vi "Configure Rx.vi"(0 "niUsrpRio Session":T3={"FPGA Interface"=refnum, "RIO Interface Number"=0, "Data Clock Rate"=0, "FPGA Data Clock Rate"=0, "Global Settings Register Bus"=refnum, "Radio 0 Settings Register Bus"=refnum, "Radio 1 Settings Register Bus"=refnum, "Radio Settings Bus Semaphore"=refnum, "DB Queues"=[], "Characterization Data Valid?"=FALSE, "EEPROM Header"={"Checksum"=0, "Product Code"=0, "Hardware Current Version"=0, "Hardware Oldest Compatible Version"=0, "EEPROM Map Current Version"=0, "EEPROM Map Oldest Compatible Version"=0, "User Password"="", "Pointer to Factory Header"=0, "Pointer to User Header"=0, "Recommended Interval"=0, "Number of Reserved Bytes"=9, "Number of Daughterboards"=0, "Daughterboard IDs"=[], "Daughterboard Serial Numbers"=[]}, "Device Data Header"={"Checksum"=0, "Number of Channels"=0, "Number of Gain Settings"=[], "Pointer to Characterization Data"=[], "Number of Reserved Bytes"=27, "Number of Frequencies"=[]}, "EEPROM Characterization Header"={"Checksum"=0, "Date"=timestamp(0 s since 1904-01-01), "Temperature"=0.0, "Misc. Info"="", "Pointer to Device Data Header"=0, "Number of Reserved Bytes"=28}, "Characterization Data"=[], "FPGA Current Version"=0, "FPGA Oldest Compatible Version"=0, "Fixed Logic Current Version"=0, "Fixed Logic Oldest Compatible Version"=0, "FPGA Radio Settings Bus Current Version"=0, "FPGA Radio Settings Bus Oldest Compatible Version"=0, "FPGA Board Config Current Version"=0, "FPGA Board Config Oldest Compatible Version"=0, "Daughterboard Clock Rate"=0, "daughterboard configuration session handles"=[]} {"Daughterboard Clock Rate" format="%#.3pHz"; "FPGA Data Clock Rate" format="%#.3pHz"; "Data Clock Rate" format="%#.3pHz"; "Characterization Data"."Frequencies [Hz]" format="%#_6p"; "EEPROM Characterization Header"."Pointer to Device Data Header" format="%x"; "EEPROM Characterization Header"."Checksum" format="%x"; "Device Data Header"."Pointer to Characterization Data" format="%x"; "Device Data Header"."Checksum" format="%x"; "EEPROM Header"."Pointer to User Header" format="%x"; "EEPROM Header"."Pointer to Factory Header" format="%x"; "EEPROM Header"."Product Code" format="%x"; "EEPROM Header"."Checksum" format="%x"}, 5 "rx config":T2={"channel configuration"=[], "transfer mode"=enum."Finite", "sample rate"=10000000.0, "number of samples"=8192, "start trigger"=enum."Immediate"} {"channel configuration"."channel configuration"."frequency" format="%#.3pHz"; "channel configuration"."channel configuration"."lo frequency" format="%#.3pHz"; "channel configuration"."channel configuration"."level" format="%#_gdBm"; "sample rate" format="%#.3pS/s"}, 7 "rx.data sink":enum16{"SFP Port 0", "SFP Port 1", "Host"}(ring)=enum."Host", 11 "error in":errorcluster) -> (4 "niUsrpRio Session (out)":T3 {"Daughterboard Clock Rate" format="%#.3pHz"; "FPGA Data Clock Rate" format="%#.3pHz"; "Data Clock Rate" format="%#.3pHz"; "Characterization Data"."Frequencies [Hz]" format="%#_6p"; "EEPROM Characterization Header"."Pointer to Device Data Header" format="%x"; "EEPROM Characterization Header"."Checksum" format="%x"; "Device Data Header"."Pointer to Characterization Data" format="%x"; "Device Data Header"."Checksum" format="%x"; "EEPROM Header"."Pointer to User Header" format="%x"; "EEPROM Header"."Pointer to Factory Header" format="%x"; "EEPROM Header"."Product Code" format="%x"; "EEPROM Header"."Checksum" format="%x"}, 6 "rx.enabled channels":string[](array[string]), 8 "vertical range":dbl[](array[numeric]) format="%#.3pVpp", 14 "rx.coerced configurations":T12 {"coerced sample rates" format="%#.3pS/s"; "coerced levels" format="%#.3gdBm"; "coerced lo frequencies" format="%#.3pHz"; "coerced frequencies" format="%#.3pHz"}, 15 "error out":errorcluster)   [LabVIEW 2018]
uses:
  <instrlib>/niUsrpRio/Config/v1/Host/Public/niUsrpRio Session.ctl
  <instrlib>/_niInstr/Register Bus/v0/Host/Public/Register Bus Session.ctl
  <instrlib>/_niInstr/Register Bus/v0/Host/Private/Session Data.ctl
  <instrlib>/niUsrpRio/Config/v1/Host/Private/DB Queue Reference.ctl
  <instrlib>/niUsrpRio/Config/v1/Host/Private/Daughterboard Data.ctl
  <instrlib>/niUsrpRio/Config/v1/Host/Private/ATR state data.ctl
  <instrlib>/niUsrpRio/Config/v1/Host/Private/Antenna Configuration.ctl
  <instrlib>/niUsrpRio/Config/v1/Host/Private/CPLD Power Mode.ctl
  <instrlib>/niUsrpRio/Config/v1/Host/Public/EEPROM Header.ctl
  <instrlib>/niUsrpRio/Config/v1/Host/Public/EEPROM Device Data Header.ctl
  <instrlib>/niUsrpRio/Config/v1/Host/Public/EEPROM Characterization Header.ctl
  <instrlib>/niUsrpRio/Config/v1/Host/Public/Characterization Data.ctl
  <instrlib>/niUsrpRio/Config/v1/Host/Public/IQ Imbalance.ctl
  Start Trigger.ctl
  Configure Signal (Level).vi
  <instrlib>/niUsrpRio/Config/v1/Host/niUsrpRio Config v1 Host.lvlib
  <instrlib>/_niInstr/Register Bus/v0/Host/niInstr Register Bus v0 Host.lvlib
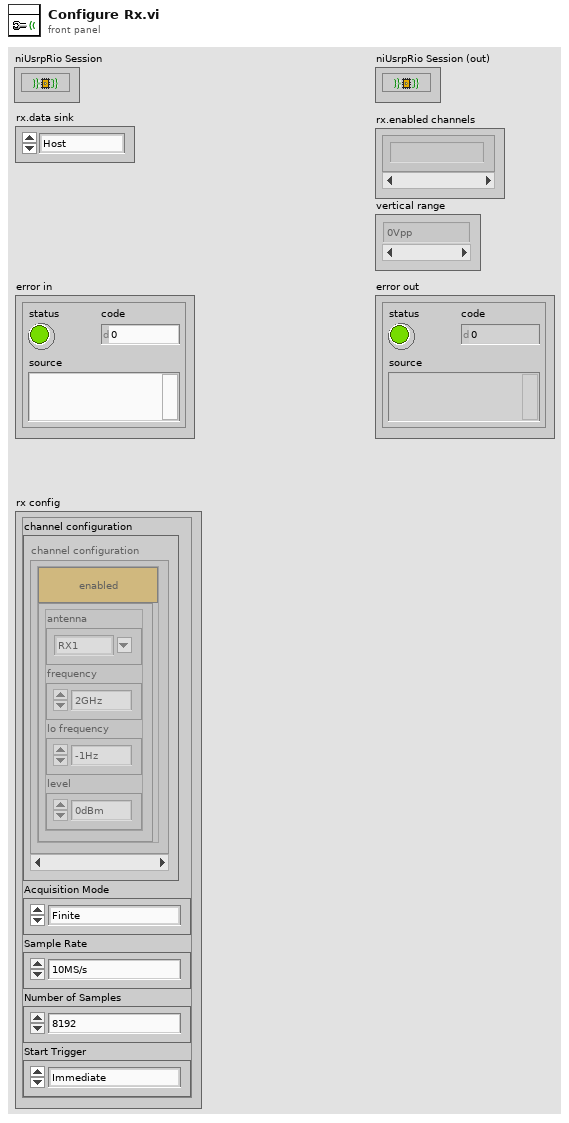
[diagram p1: front panel]
types:
  T1 = typedef "Start Trigger.ctl" = enum8{"Software", "Digital Edge", "Rx Start Trigger", "Tx Start Trigger", "Immediate", "Future Time Event"}
  T2 = cluster{"channel configuration":cluster{"channel enable":bool, "channel configuration":cluster{"antenna":string, "frequency":dbl, "lo frequency":dbl, "level":dbl}}[], "transfer mode":enum16{"Finite", "Continuous"}, "sample rate":dbl, "number of samples":u32, "start trigger":T1}
  T3 = typedef "niUsrpRio Config v1 Host.lvlib/niUsrpRio Session.ctl" = cluster{"FPGA Interface":refnum<k20>, "RIO Interface Number":u32, "Data Clock Rate":u32, "FPGA Data Clock Rate":u32, "Global Settings Register Bus":T4, "Radio 0 Settings Register Bus":T4, "Radio 1 Settings Register Bus":T4, "Radio Settings Bus Semaphore":T5, "DB Queues":T6[], "Characterization Data Valid?":bool, "EEPROM Header":T7, "Device Data Header":T8, "EEPROM Characterization Header":T9, "Characterization Data":T10[], "FPGA Current Version":u32, "FPGA Oldest Compatible Version":u32, "Fixed Logic Current Version":u32, "Fixed Logic Oldest Compatible Version":u32, "FPGA Radio Settings Bus Current Version":u32, "FPGA Radio Settings Bus Oldest Compatible Version":u32, "FPGA Board Config Current Version":u32, "FPGA Board Config Oldest Compatible Version":u32, "Daughterboard Clock Rate":u32, "daughterboard configuration session handles":u64[]}
  T4 = typedef "niInstr Register Bus v0 Host.lvlib/Register Bus Session.ctl" = refnum<queue>
  T5 = typedef "Semaphore RefNum" = refnum<k1>
  T6 = typedef "niUsrpRio Config v1 Host.lvlib/DB Queue Reference.ctl" = refnum<queue>
  T7 = typedef "niUsrpRio Config v1 Host.lvlib/EEPROM Header.ctl" = cluster{"Checksum":u32, "Product Code":u16, "Hardware Current Version":u16, "Hardware Oldest Compatible Version":u16, "EEPROM Map Current Version":u16, "EEPROM Map Oldest Compatible Version":u16, "User Password":string, "Pointer to Factory Header":u32, "Pointer to User Header":u32, "Recommended Interval":u16, "Number of Reserved Bytes":i32, "Number of Daughterboards":u8, "Daughterboard IDs":u16[], "Daughterboard Serial Numbers":string[]}
  T8 = typedef "niUsrpRio Config v1 Host.lvlib/EEPROM Device Data Header.ctl" = cluster{"Checksum":u32, "Number of Channels":u8, "Number of Gain Settings":u16[], "Pointer to Characterization Data":u32[], "Number of Reserved Bytes":i32, "Number of Frequencies":u16[]}
  T9 = typedef "niUsrpRio Config v1 Host.lvlib/EEPROM Characterization Header.ctl" = cluster{"Checksum":u32, "Date":timestamp, "Temperature":sgl, "Misc. Info":string, "Pointer to Device Data Header":u32, "Number of Reserved Bytes":i32}
  T10 = typedef "niUsrpRio Config v1 Host.lvlib/Characterization Data.ctl" = cluster{"Gains[dB]":dbl[], "Frequencies [Hz]":dbl[], "IQ Imbalance Table":T11[], "Measured Gains[dB]":dbl[][]}
  T11 = typedef "niUsrpRio Config v1 Host.lvlib/IQ Imbalance.ctl" = cluster{"Gain Imbalance [linear]":dbl, "Phase Imbalance [radians]":dbl, "Offset":cdb}
  T12 = cluster{"coerced frequencies":dbl[], "coerced lo frequencies":dbl[], "coerced levels":dbl[], "coerced sample rates":dbl[]}
  T13 = cluster{"channel enable":bool, "channel configuration":cluster{"antenna":string, "frequency":dbl, "lo frequency":dbl, "level":dbl}}[]
  T14 = cluster{"antenna":string, "frequency":dbl, "lo frequency":dbl, "level":dbl}[]
  T15 = typedef "niUsrpRio Config v1 Host.lvlib/DB Types.ctl" = enum16{"sbx", "cbx", "wbx", "unknown", "ubx", "twinrx"}
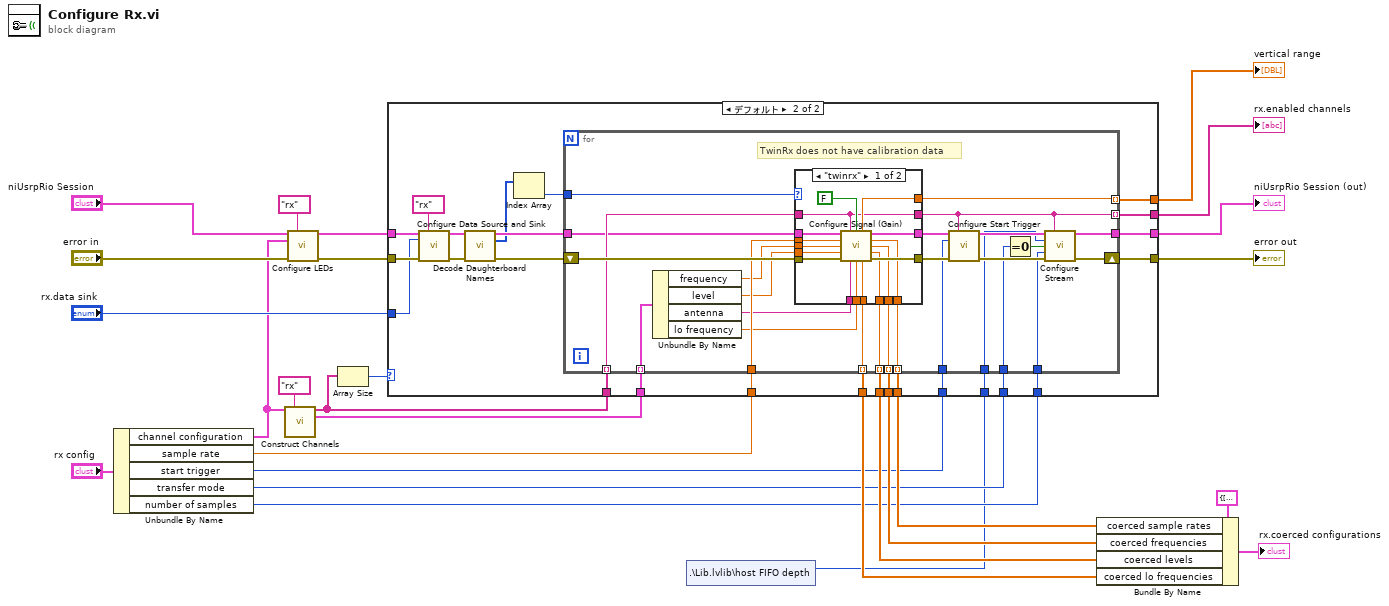
[diagram p0: block diagram]
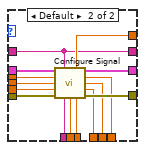
[diagram p3: hidden frame]
diagram:
  n1 = Unbundle By Name("rx config") -> ("channel configuration"=w2:T13, "sample rate"=w11:dbl, "start trigger"=w10:T1, "transfer mode"=w8:enum16{"Finite", "Continuous"}, "number of samples"=w9:u32)
  n2 = call "Construct Channels.vi"("channel configurations"=w2, "scope"="rx") -> ("enabled channels"=w14:string[], "enabled channel configurations"=w20:T14)  [unwired: 12 in]
  n3 = call "Configure LEDs.vi"("niUsrpRio Session"="niUsrpRio Session", "scope"="rx", "channel configurations"=w2, "error in"="error in") -> ("niUsrpRio Session (out)"=w5:T3, "error out"=w4:errorcluster)  [unwired: 10 in]
  n4 = Array Size(array=w14) -> (size(s)=w15:i32)
  n5 = shared-variable ".\\Lib.lvlib\\host FIFO depth"() -> (w1:u32)  [unwired: 1 in, 1 out]
  n6 = case shown="デフォルト" w15 {
    tunnel: [_ w54] -> w27
    tunnel: [_ w53] -> w26
    tunnel: [_ w52] -> w25
    tunnel: [_ w51] -> w24
    tunnel: [w29 w50] -> w23
    tunnel: [w28 w49] -> w22
    tunnel: w20 -> [_ w48]
    tunnel: [_ w47] -> w19
    tunnel: [_ w46] -> w16
    tunnel: w11 -> [_ w45]
    tunnel: w10 -> [_ w44]
    tunnel: w8 -> [_ w43]
    tunnel: w9 -> [_ w42]
    tunnel: w4 -> [w28 w40]
    tunnel: w5 -> [w29 w37]
    tunnel: w14 -> [_ w41]
    tunnel: "rx.data sink" -> [_ w39]
    tunnel: w1 -> [_ w30]
    frame 0 {
    }
    frame Default {
      n7 = call "Configure Data Source and Sink.vi"("niUsrpRio Session"=w37, "scope"="rx", "data stream config"=w39, "error in"=w40) -> ("niUsrpRio Session (out)"=w36:T3, "error out"=w35:errorcluster)  [unwired: 10 in]
      n8 = call <instrlib>:"Decode Daughterboard Names.vi"("niUsrpRio Session"=w36, "error in"=w35) -> ("niUsrpRio Session (out)"=w34:T3, "daughterboard names"=w32:T15[], "error out"=w33:errorcluster)  [unwired: 10 in, 1 out]
      n9 = Index Array(array=w32) -> (element=w31:T15)  [unwired: 1 in]
      n10 = for "channel configuration" {
        tunnel: [w78] -> w50
        shift-right: [w79] -> w49
        shift-left: w33 -> [w71]
        tunnel: w41 -> [w60] mode=indexing
        tunnel: w48 -> [w77] mode=indexing
        tunnel: [w72] -> w47 mode=indexing
        tunnel: [w76] -> w54 mode=indexing
        tunnel: [w75] -> w53 mode=indexing
        tunnel: [w74] -> w52 mode=indexing
        tunnel: [w73] -> w51 mode=indexing
        tunnel: [w57] -> w46 mode=indexing
        tunnel: w45 -> [w70]
        tunnel: w44 -> [w69]
        tunnel: w43 -> [w68]
        tunnel: w42 -> [w67]
        tunnel: w34 -> [w58]
        tunnel: w31 -> [w56]
        tunnel: w30 -> [w55]
        # "TwinRx does not have calibration data"
        n11 = Unbundle By Name(w77) -> ("frequency"=w64:dbl, "level"=w63:dbl, "antenna"=w62:string, "lo frequency"=w61:dbl)
        n12 = case shown="\"twinrx\"" w56 {
          tunnel: [w89 w112] -> w80
          tunnel: [w83 w111] -> w76
          tunnel: [w84 w110] -> w75
          tunnel: [w85 w109] -> w74
          tunnel: [w90 w108] -> w73
          tunnel: [w87 w107] -> w72
          tunnel: w71 -> [w93 w106]
          tunnel: w70 -> [w96 w105]
          tunnel: [w88 w104] -> w65
          tunnel: w64 -> [w95 w103]
          tunnel: w63 -> [w94 w102]
          tunnel: w62 -> [w92 w101]
          tunnel: w61 -> [w91 w100]
          tunnel: w60 -> [w82 w98]
          tunnel: w58 -> [w97 w99]
          tunnel: [w82 w98] -> w57
          frame "twinrx" {
            n13 = call "Configure Signal (Gain).vi"("niUsrpRio Session"=w97, "scope"=w82, "Correct Impairments?"=FALSE, "sample rate [S/s]"=w96, "frequency [Hz]"=w95, "gain [dB]"=w94, "error in"=w93, "Active Antenna"=w92, "LO frequency [Hz]"=w91) -> ("cumulative digital gain"=w87:dbl, "niUsrpRio Session (out)"=w88:T3, "coerced sample rate [S/s]"=w83:dbl, "coerced frequency [Hz]"=w84:dbl, "coerced gain [dB]"=w85:dbl, "coerced LO frequency [Hz]"=w90:dbl, "error out"=w89:errorcluster)
          }
          frame Default {
            n14 = call-poly "Configure Signal.vi"("niUsrpRio Session"=w99, "scope"=w98, "sample rate [S/s]"=w105, "frequency [Hz]"=w103, "level [dBm]"=w102, "error in"=w106, "Active Antenna"=w101, "LO frequency [Hz]"=w100) -> ("coerced vertical range [Vpp]"=w107:dbl, "niUsrpRio Session (out)"=w104:T3, "coerced sample rate [S/s]"=w111:dbl, "coerced frequency [Hz]"=w110:dbl, "coerced level [dBm]"=w109:dbl, "coerced LO frequency [Hz]"=w108:dbl, "error out"=w112:errorcluster)  [unwired: 1 in]
          }
        }
        n15 = call "Configure Start Trigger.vi"("niUsrpRio Session"=w65, "scope"=w57, "start trigger"=w69, "error in"=w80) -> ("niUsrpRio Session (out)"=w66:T3, "error out"=w81:errorcluster)  [unwired: 10 in]
        n16 = Equal To 0?(x=w68) -> (x = 0?=w59:bool)
        n17 = call "Configure Stream.vi"("niUsrpRio Session"=w66, "scope"=w57, "host FIFO depth"=w55, "number of samples is finite"=w59, "number of samples"=w67, "error in"=w81) -> ("niUsrpRio Session (out)"=w78:T3, "error out"=w79:errorcluster)  [unwired: 8 in]
      }
    }
  }
  "niUsrpRio Session (out)" <- w23
  "error out" <- w22
  "vertical range" <- w19
  "rx.enabled channels" <- w16
  n18 = Bundle By Name(cluster=T12 {"coerced frequencies"=[], "coerced lo frequencies"=[], "coerced levels"=[], "coerced sample rates"=[]} ("coerced configurations"), "coerced sample rates"=w27, "coerced frequencies"=w26, "coerced levels"=w25, "coerced lo frequencies"=w24) -> (→"rx.coerced configurations":T12)
